vi "configure Measurement Hioky.vi"(6 "Enable Auto Range (T: Enable)":bool=TRUE, 7 "Mode clamp(only use with clamp measurement)":string(combo)="9010", 8 "error in (no error)":errorcluster, 9 "Manual Range (1.00)":dbl=1.0 format="%_3f", 10 "Function (0: DC Voltage)":u16(ring) items=["DC Voltage", "AC Voltage", "2 - Wire Resistance", "2 -Wire Resistance low power", "4 - Wire Resistance", "4- Wire Resistance low power", "DC Current", "AC Current", "CLAMP DC", "CLAMP AC", "Frequency", "Continuity", "Diode Checking"], 11 "VISA resource name":refnum<visa-resource-name>) -> (0 "error out":errorcluster, 3 "VISA resource name out":refnum<visa-resource-name>)   [LabVIEW 2017]
panel:
  # "AUTO RANGE IN ONLY FOR VOLT,CURRENT, RESISTANCE MEASUREMENT"
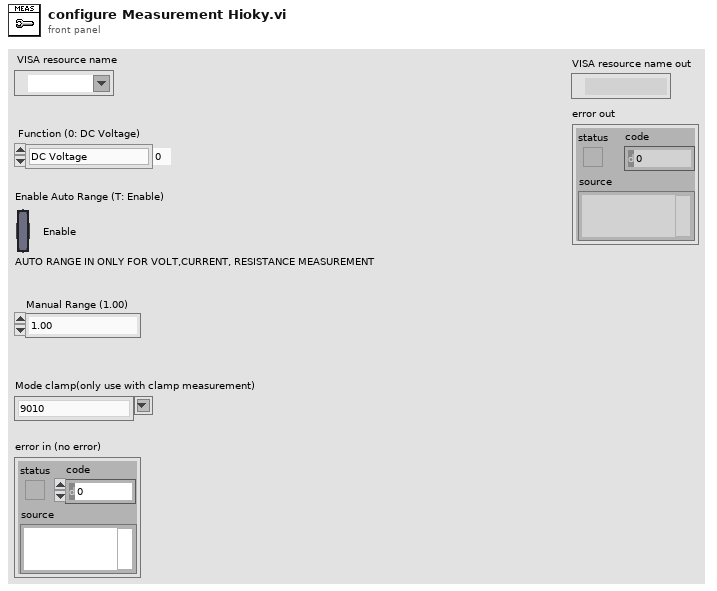
[diagram p1: front panel]
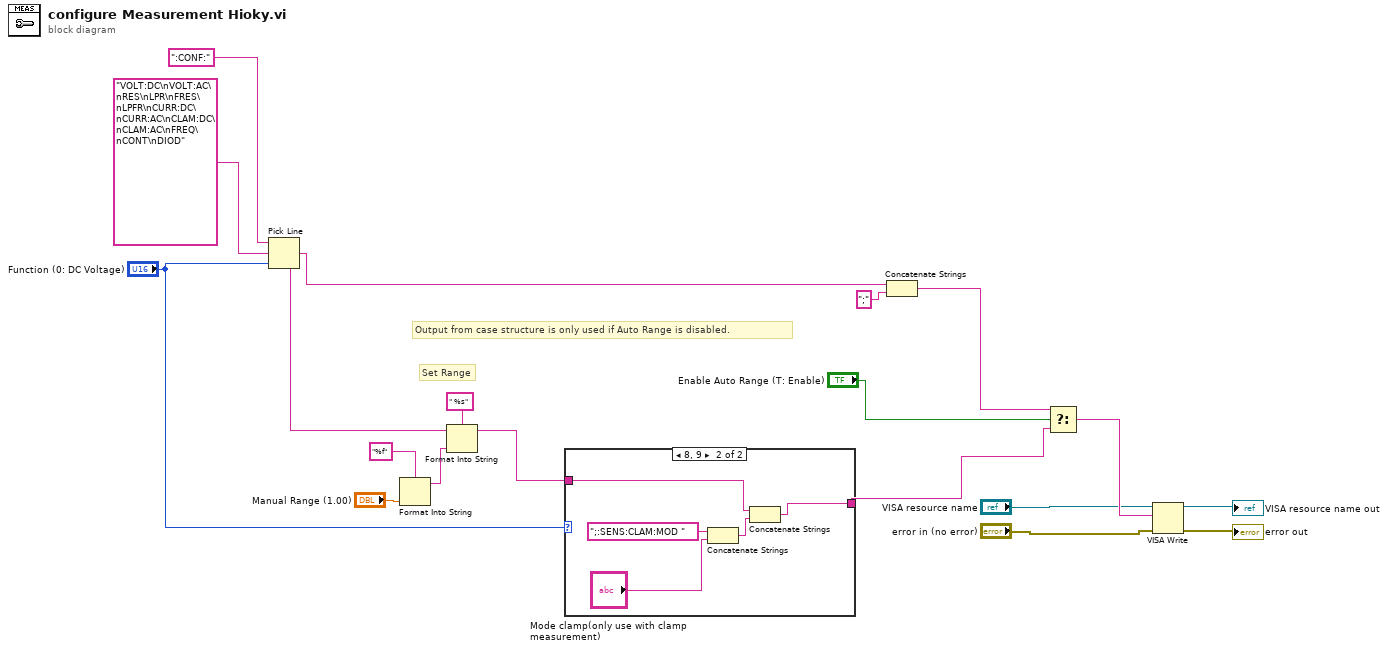
[diagram p0: block diagram]
diagram:
  # "Set Range"
  # "Output from case structure is only used if Auto Range is disabled."
  n1 = Pick Line(string ("")=":CONF:", multi-line string="VOLT:DC\nVOLT:AC\nRES\nLPR\nFRES\nLPFR\nCURR:DC\nCURR:AC\nCLAM:DC\nCLAM:AC\nFREQ\nCONT\nDIOD", line index="Function (0: DC Voltage)") -> (output string=w3:string)
  n2 = Format Into String(format string="%f", "Manual Range (1.00)") -> (resulting string=w7:string)  [unwired: 2 in, 1 out]
  n3 = Format Into String(format string=" %s", initial string=w3, w7) -> (resulting string=w5:string)  [unwired: 1 in, 1 out]
  n4 = case shown="8, 9" "Function (0: DC Voltage)" {
    tunnel: [w19 w20] -> w6
    tunnel: w5 -> [w19 w24]
    frame Default {
    }
    frame 8, 9 {
      n5 = Concatenate Strings(";:SENS:CLAM:MOD " ("string"), "Mode clamp(only use with clamp measurement)") -> (w21:string)
      n6 = Concatenate Strings(w24, w21) -> (w20:string)
    }
  }
  n7 = Concatenate Strings(w3, ";" ("t")) -> (w2:string)
  n8 = Select(t=w2, s="Enable Auto Range (T: Enable)", f=w6) -> (s? t:f=w18:string)
  n9 = VISA Write(VISA resource name="VISA resource name", write buffer=w18, error in (no error)="error in (no error)") -> (VISA resource name out=→"VISA resource name out":refnum<visa-resource-name>, error out=→"error out":errorcluster)  [unwired: 1 out]
